vi "Get Paths.vi"(8 "error in (no error)":errorcluster) -> (0 "error out":errorcluster, 1 "Image URL":string, 2 "Root folder":path, 3 "Image folder":path)   [LabVIEW 2017, in "Front Panel Publisher.lvlib" / "Front Panel Manager.lvclass"]
uses:
  Front Panel Manager.lvclass
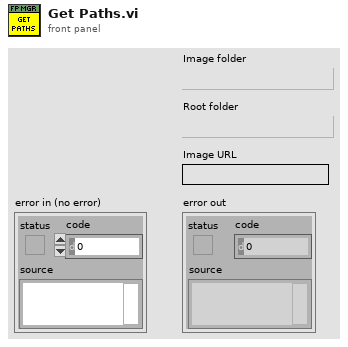
[diagram p1: front panel]
types:
  T1 = typedef "Front Panel Publisher.lvlib/Front Panel Manager.lvclass/Object Attributes.ctl" = cluster{"WebFrontPanels":refnum<class "Web Front Panel.lvclass">[], "WFP Names":string[], "Root folder":path, "Websocket Info":T2}
  T2 = typedef "Front Panel Publisher.lvlib/Front Panel Manager.lvclass/Websocket Info.ctl" = cluster{"Hostname":string, "Port":u16}
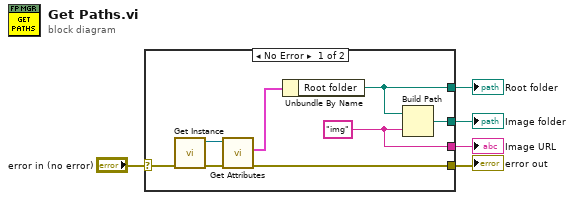
[diagram p0: block diagram]
diagram:
  n1 = case shown="No Error" "error in (no error)" {
    selector: "error in (no error)" -> [w10 w14]
    tunnel: [w12 w14] -> w4
    tunnel: [w8 _] -> w3
    tunnel: [w7 _] -> w2
    tunnel: [w6 _] -> w1
    frame No Error {
      w6 = "img" ("name or relative path")
      n2 = call "Get Instance.vi"("error in (no error)"=w10) -> ("error out"=w9:errorcluster, "FP Manager Out"=w11:refnum<class "Front Panel Manager.lvclass">)  [unwired: 6 in, 3 out]
      n3 = call "Get Attributes.vi"("error in (no error)"=w9, "FP Management In"=w11) -> ("error out"=w12:errorcluster, "Data"=w13:T1)  [unwired: 6 in, 2 out]
      n4 = Unbundle By Name(w13) -> ("Root folder"=w8:path)
      n5 = Build Path(base path=w8, name or relative path=w6) -> (appended path=w7:path)
    }
    frame Error {
    }
  }
  "error out" <- w4
  "Root folder" <- w3
  "Image folder" <- w2
  "Image URL" <- w1
